vi "Initiate and Fetch Time (Multi).vi"(0 "niUsrpRio Sessions":T3[](array[typedef]) {"Daughterboard Clock Rate" format="%#.3pHz"; "FPGA Data Clock Rate" format="%#.3pHz"; "Data Clock Rate" format="%#.3pHz"; "Characterization Data"."Frequencies [Hz]" format="%#_6p"; "EEPROM Characterization Header"."Pointer to Device Data Header" format="%x"; "EEPROM Characterization Header"."Checksum" format="%x"; "Device Data Header"."Pointer to Characterization Data" format="%x"; "Device Data Header"."Checksum" format="%x"; "EEPROM Header"."Pointer to User Header" format="%x"; "EEPROM Header"."Pointer to Factory Header" format="%x"; "EEPROM Header"."Product Code" format="%x"; "EEPROM Header"."Checksum" format="%x"}, 1 "rx channels":T1[](array[typedef]) {"rx.coerced configurations"."coerced sample rates" format="%#.3pS/s"; "rx.coerced configurations"."coerced levels" format="%#.3gdBm"; "rx.coerced configurations"."coerced lo frequencies" format="%#.3pHz"; "rx.coerced configurations"."coerced frequencies" format="%#.3pHz"; "rx config"."channel configuration"."channel configuration"."frequency" format="%#.3pHz"; "rx config"."channel configuration"."channel configuration"."lo frequency" format="%#.3pHz"; "rx config"."channel configuration"."channel configuration"."level" format="%#_gdBm"; "rx config"."sample rate" format="%#.3pS/s"; "vertical range" format="%#.3pVpp"}, 5 "first iteration":bool, 7 "start trigger time":timestamp, 11 "error in":errorcluster, 12 "leading samples to trim":u32) -> (4 "niUsrpRio Sessions (out)":T3[](array[typedef]) {"Daughterboard Clock Rate" format="%#.3pHz"; "FPGA Data Clock Rate" format="%#.3pHz"; "Data Clock Rate" format="%#.3pHz"; "Characterization Data"."Frequencies [Hz]" format="%#_6p"; "EEPROM Characterization Header"."Pointer to Device Data Header" format="%x"; "EEPROM Characterization Header"."Checksum" format="%x"; "Device Data Header"."Pointer to Characterization Data" format="%x"; "Device Data Header"."Checksum" format="%x"; "EEPROM Header"."Pointer to User Header" format="%x"; "EEPROM Header"."Pointer to Factory Header" format="%x"; "EEPROM Header"."Product Code" format="%x"; "EEPROM Header"."Checksum" format="%x"}, 6 "complex baseband data":waveform(cdb)[](array[waveform]), 10 "elements in fifo":u32[](array[numeric]), 15 "error out":errorcluster)   [LabVIEW 2020]
doc: "Initiates acquisition and then fetches data from the device.\n\nVIs that must execute before this VI:\nOpen and Configure.vi\n\n<B>Input Parameters</B>\n\n<B>niUsrpRio Session</B> is the object created by the Open VI and used as the session handle for the USRP RIO design library.\n\n<B>first iteration</B> is used to determine if the device needs to be triggered. If this VI is in a loop, wire the iteration count to Equals Zero and then to this terminal. If this VI is not in a loop, wire a TRUE constant to this this terminal.\n\n<B>start trigger time</B> specifies the absolute time to initiate the start trigger. Only applies when the start trigger is set to Future Event.\n\n<B>error in</B> describes error conditions that occur before this node runs. This input provides standard 'error in' functionality.\n\n<B>Output Parameters</B>\n\n<B>niUsrpRio Session (out)</B> is the niUsrpRio session used in all subsequent USRP RIO design library host VIs.\n\n<B>complex baseband data</B> received by the device.\n\n<B>error out</B> contains error information. This output provides standard 'error out' functionality."
uses:
  <instrlib>/niUsrpRio/Config/v1/Host/Public/niUsrpRio Session.ctl
  <instrlib>/_niInstr/Register Bus/v0/Host/Public/Register Bus Session.ctl
  <instrlib>/_niInstr/Register Bus/v0/Host/Private/Session Data.ctl
  <instrlib>/niUsrpRio/Config/v1/Host/Private/DB Queue Reference.ctl
  <instrlib>/niUsrpRio/Config/v1/Host/Private/Daughterboard Data.ctl
  <instrlib>/niUsrpRio/Config/v1/Host/Private/ATR state data.ctl
  <instrlib>/niUsrpRio/Config/v1/Host/Private/Antenna Configuration.ctl
  <instrlib>/niUsrpRio/Config/v1/Host/Private/CPLD Power Mode.ctl
  <instrlib>/niUsrpRio/Config/v1/Host/Public/EEPROM Header.ctl
  <instrlib>/niUsrpRio/Config/v1/Host/Public/EEPROM Device Data Header.ctl
  <instrlib>/niUsrpRio/Config/v1/Host/Public/EEPROM Characterization Header.ctl
  <instrlib>/niUsrpRio/Config/v1/Host/Public/Characterization Data.ctl
  <instrlib>/niUsrpRio/Config/v1/Host/Public/IQ Imbalance.ctl
  Rx Channels.ctl
  Start Trigger.ctl
  Fetch Rx Data (CDB WDT).vi
  <instrlib>/_niInstr/Register Bus/v0/Host/niInstr Register Bus v0 Host.lvlib
  <instrlib>/niUsrpRio/Config/v1/Host/niUsrpRio Config v1 Host.lvlib
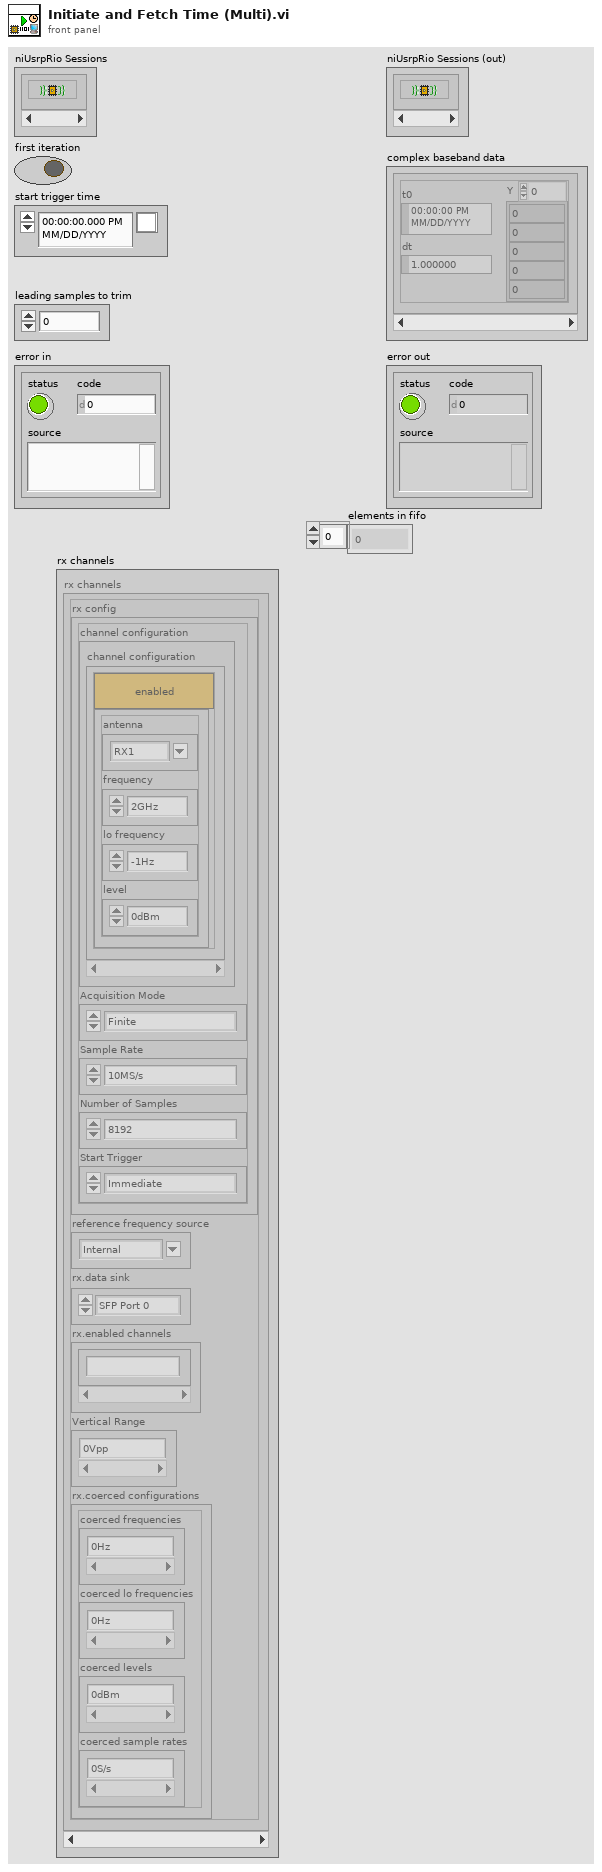
[diagram p1: front panel]
types:
  T1 = typedef "Rx Channels.ctl" = cluster{"rx config":cluster{"channel configuration":cluster{"channel enable":bool, "channel configuration":cluster{"antenna":string, "frequency":dbl, "lo frequency":dbl, "level":dbl}}[], "transfer mode":enum16{"Finite", "Continuous"}, "sample rate":dbl, "number of samples":u32, "start trigger":T2}, "reference frequency source":string, "rx.data sink":enum16{"SFP Port 0", "SFP Port 1", "Host"}, "rx.enabled channels":string[], "vertical range":dbl[], "rx.coerced configurations":cluster{"coerced frequencies":dbl[], "coerced lo frequencies":dbl[], "coerced levels":dbl[], "coerced sample rates":dbl[]}}
  T2 = typedef "Start Trigger.ctl" = enum8{"Software", "Digital Edge", "Rx Start Trigger", "Tx Start Trigger", "Immediate", "Future Time Event"}
  T3 = typedef "niUsrpRio Config v1 Host.lvlib/niUsrpRio Session.ctl" = cluster{"FPGA Interface":refnum<k20>, "RIO Interface Number":u32, "Data Clock Rate":u32, "FPGA Data Clock Rate":u32, "Global Settings Register Bus":T4, "Radio 0 Settings Register Bus":T4, "Radio 1 Settings Register Bus":T4, "Radio Settings Bus Semaphore":T5, "DB Queues":T6[], "Characterization Data Valid?":bool, "EEPROM Header":T7, "Device Data Header":T8, "EEPROM Characterization Header":T9, "Characterization Data":T10[], "FPGA Current Version":u32, "FPGA Oldest Compatible Version":u32, "Fixed Logic Current Version":u32, "Fixed Logic Oldest Compatible Version":u32, "FPGA Radio Settings Bus Current Version":u32, "FPGA Radio Settings Bus Oldest Compatible Version":u32, "FPGA Board Config Current Version":u32, "FPGA Board Config Oldest Compatible Version":u32, "Daughterboard Clock Rate":u32, "daughterboard configuration session handles":u64[]}
  T4 = typedef "niInstr Register Bus v0 Host.lvlib/Register Bus Session.ctl" = refnum<queue>
  T5 = typedef "Semaphore RefNum" = refnum<k1>
  T6 = typedef "niUsrpRio Config v1 Host.lvlib/DB Queue Reference.ctl" = refnum<queue>
  T7 = typedef "niUsrpRio Config v1 Host.lvlib/EEPROM Header.ctl" = cluster{"Checksum":u32, "Product Code":u16, "Hardware Current Version":u16, "Hardware Oldest Compatible Version":u16, "EEPROM Map Current Version":u16, "EEPROM Map Oldest Compatible Version":u16, "User Password":string, "Pointer to Factory Header":u32, "Pointer to User Header":u32, "Recommended Interval":u16, "Number of Reserved Bytes":i32, "Number of Daughterboards":u8, "Daughterboard IDs":u16[], "Daughterboard Serial Numbers":string[]}
  T8 = typedef "niUsrpRio Config v1 Host.lvlib/EEPROM Device Data Header.ctl" = cluster{"Checksum":u32, "Number of Channels":u8, "Number of Gain Settings":u16[], "Pointer to Characterization Data":u32[], "Number of Reserved Bytes":i32, "Number of Frequencies":u16[]}
  T9 = typedef "niUsrpRio Config v1 Host.lvlib/EEPROM Characterization Header.ctl" = cluster{"Checksum":u32, "Date":timestamp, "Temperature":sgl, "Misc. Info":string, "Pointer to Device Data Header":u32, "Number of Reserved Bytes":i32}
  T10 = typedef "niUsrpRio Config v1 Host.lvlib/Characterization Data.ctl" = cluster{"Gains[dB]":dbl[], "Frequencies [Hz]":dbl[], "IQ Imbalance Table":T11[], "Measured Gains[dB]":dbl[][]}
  T11 = typedef "niUsrpRio Config v1 Host.lvlib/IQ Imbalance.ctl" = cluster{"Gain Imbalance [linear]":dbl, "Phase Imbalance [radians]":dbl, "Offset":cdb}
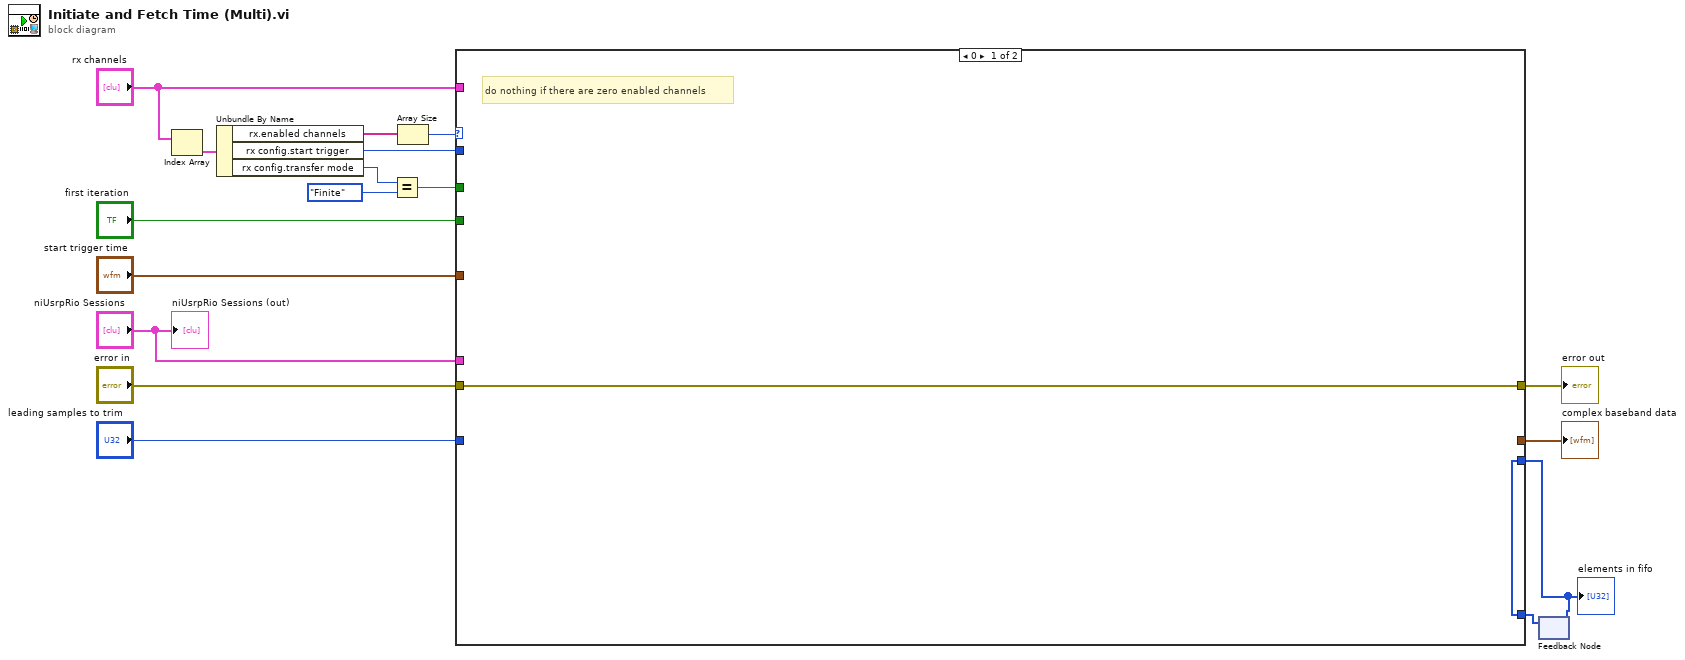
[diagram p0: block diagram]
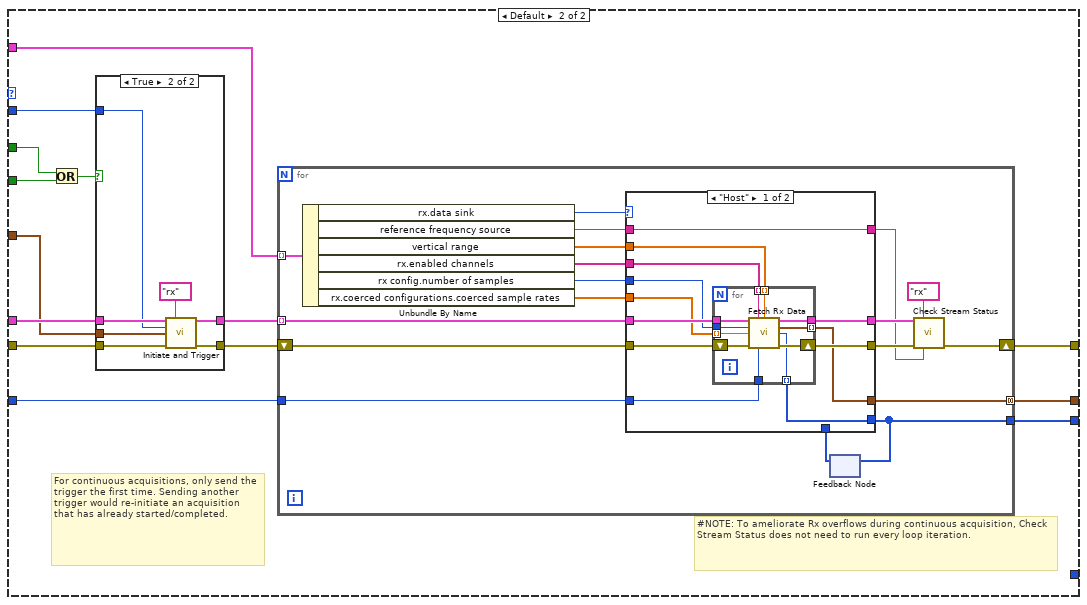
[diagram p2: hidden frame]
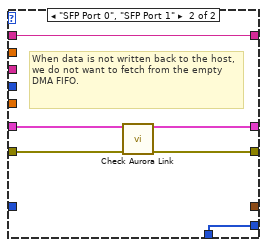
[diagram p4: hidden frame]
diagram:
  n1 = Index Array(array="rx channels") -> (element=w13:T1)  [unwired: 1 in]
  n2 = Unbundle By Name(w13) -> ("rx.enabled channels"=w10:string[], "rx config.start trigger"=w12:T2, "rx config.transfer mode"=w5:enum16{"Finite", "Continuous"})
  n3 = Equal?(x=w5, y=enum16{"Finite", "Continuous"}."Finite" ("x")) -> (x = y?=w3:bool)
  n4 = Array Size(array=w10) -> (size(s)=w9:i32)
  n5 = feedback #1() -> (w1:u32[])  [unwired: 1 in]
  n6 = case shown="0" w9 {
    tunnel: "niUsrpRio Sessions" -> [_ w32]
    tunnel: "error in" -> [w19 w31]
    tunnel: "first iteration" -> [_ w22]
    tunnel: [w19 w29] -> w14
    tunnel: "start trigger time" -> [_ w21]
    tunnel: w12 -> [_ w27]
    tunnel: w3 -> [_ w26]
    tunnel: "rx channels" -> [_ w25]
    tunnel: "leading samples to trim" -> [_ w24]
    tunnel: [_ w23] -> w17
    tunnel: [w18 w20] -> w2
    tunnel: w1 -> [w18 _]
    frame 0 {
      # "do nothing if there are zero enabled channels"
    }
    frame Default {
      # "#NOTE: To ameliorate Rx overflows during continuous acquisition, Check Stream Status does not need to run every loop iteration."
      # "For continuous acquisitions, only send the trigger the first time. Sending another trigger would re-initiate an acquisition that has already started/completed."
      n7 = Or(x=w26, y=w22) -> (x .or. y?=w33:bool)
      n8 = case shown="True" w33 {
        tunnel: w31 -> [w35 w41]
        tunnel: [w35 w39] -> w28
        tunnel: w32 -> [w34 w42]
        tunnel: [w34 w40] -> w30
        tunnel: w27 -> [_ w38]
        tunnel: w21 -> [_ w36]
        frame False {
        }
        frame True {
          n9 = call "Initiate and Trigger.vi"("niUsrpRio Sessions"=w42, "scope"="rx", "start trigger"=w38, "start trigger time"=w36, "error in"=w41) -> ("niUsrpRio Sessions (out)"=w40:T3[], "error out"=w39:errorcluster)  [unwired: 9 in]
        }
      }
      n10 = for {
        shift-right: [w58] -> w29
        shift-left: w28 -> [w57]
        tunnel: w30 -> [w56] mode=indexing
        tunnel: w25 -> [w55] mode=indexing
        tunnel: w24 -> [w51]
        tunnel: [w49] -> w23 mode=concatenating
        tunnel: [w44] -> w20
        n11 = Unbundle By Name(w55) -> ("rx.data sink"=w45:enum16{"SFP Port 0", "SFP Port 1", "Host"}, "reference frequency source"=w47:string, "vertical range"=w53:dbl[], "rx.enabled channels"=w54:string[], "rx config.number of samples"=w52:u32, "rx.coerced configurations.coerced sample rates"=w48:dbl[])
        n12 = feedback #2() -> (w43:u32[])  [unwired: 1 in]
        n13 = case shown="\"Host\"" w45 {
          tunnel: [w72 w86] -> w60
          tunnel: [w71 w87] -> w59
          tunnel: w57 -> [w70 w88]
          tunnel: w56 -> [w69 w85]
          tunnel: w54 -> [w68 _]
          tunnel: w53 -> [w67 _]
          tunnel: w52 -> [w66 _]
          tunnel: w51 -> [w65 _]
          tunnel: [w64 _] -> w49
          tunnel: w48 -> [w63 _]
          tunnel: w47 -> [w62 w89]
          tunnel: [w62 w89] -> w46
          tunnel: [w61 w84] -> w44
          tunnel: w43 -> [_ w84]
          frame "Host" {
            n14 = for {
              shift-right: [w80] -> w71
              shift-left: w70 -> [w82]
              tunnel: w68 -> [w79] mode=indexing
              tunnel: w67 -> [w78] mode=indexing
              tunnel: w69 -> [w83]
              tunnel: [w81] -> w72
              tunnel: w66 -> [w77]
              tunnel: w65 -> [w75]
              tunnel: [w76] -> w64 mode=indexing
              tunnel: w63 -> [w74] mode=indexing
              tunnel: [w73] -> w61 mode=indexing
              n15 = call-poly "Fetch Rx Data.vi"("niUsrpRio Session"=w83, "scope"=w79, "vertical range"=w78, "number of samples"=w77, "sample rate"=w74, "error in"=w82, "leading samples to trim"=w75) -> ("niUsrpRio Session (out)"=w81:T3, "Waveform"=w76:waveform(cdb), "Elements Remaining"=w73:u32, "error out"=w80:errorcluster)  [unwired: 5 in]
            }
          }
          frame "SFP Port 0", "SFP Port 1" {
            # "When data is not written back to the host, we do not want to fetch from the empty DMA FIFO."
            n16 = call "Check Aurora Link.vi"("niUsrpRio Session"=w85, "error in"=w88) -> ("niUsrpRio Session (out)"=w86:T3, "error out"=w87:errorcluster)  [unwired: 12 in]
          }
        }
        n17 = feedback-in #2(w44) -> ()
        n18 = call "Check Stream Status.vi"("niUsrpRio Session"=w60, "scope"="rx", "error in"=w59, "reference frequency source"=w46) -> ("error out"=w58:errorcluster)  [unwired: 9 in, 2 out]
      }
    }
  }
  "error out" <- w14
  "complex baseband data" <- w17
  "elements in fifo" <- w2
  n19 = feedback-in #1(w2) -> ()
  "niUsrpRio Sessions (out)" <- "niUsrpRio Sessions"
